vi "DigitalReadDigitalWrite.vi"() -> ()   [LabVIEW 2015]
panel:
  out "YLDRMErrorOut":errorcluster
  out "YLDRMPortOut":refnum<visa-resource-name>
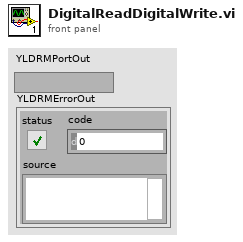
[diagram p1: front panel]
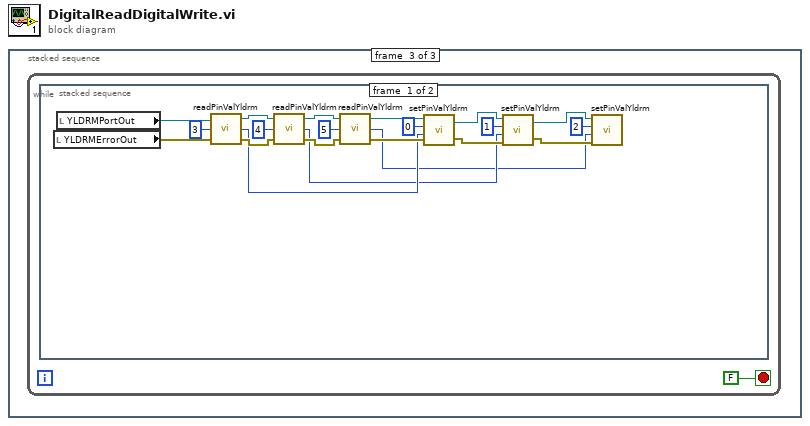
[diagram p0: block diagram]
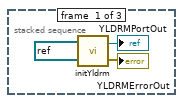
[diagram p2: hidden frame]
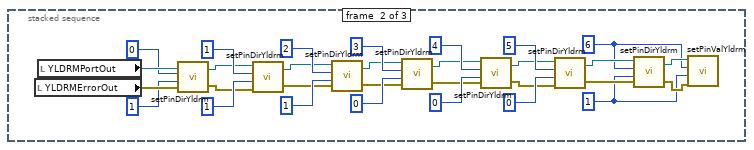
[diagram p3: hidden frame]
diagram:
  n1 = stacked-sequence {
    frame #0 {
      n2 = call "initYldrm.vi"("YLDRMPortInp"=refnum<visa-resource-name> "COM9") -> ("YLDRMPortOut"=→"YLDRMPortOut":refnum<visa-resource-name>, "YLDRMErrorOut"=→"YLDRMErrorOut":errorcluster)
    }
    frame #1 {
      w4 = u8 1 ("dir")
      w5 = u8 6 ("pin")
      n3 = local read "YLDRMErrorOut"() -> (w32:errorcluster)
      n4 = local read "YLDRMPortOut"() -> (w33:refnum<visa-resource-name>)
      n5 = call "setPinDirYldrm.vi"("YLDRMErrorInp"=w32, "dir"=u8 1, "pin"=u8 0, "YLDRMPortInp"=w33) -> ("YLDRMErrorOut"=w13:errorcluster, "YLDRMPortOut"=w19:refnum<visa-resource-name>)
      n6 = call "setPinDirYldrm.vi"("YLDRMErrorInp"=w13, "dir"=u8 1, "pin"=u8 1, "YLDRMPortInp"=w19) -> ("YLDRMErrorOut"=w12:errorcluster, "YLDRMPortOut"=w18:refnum<visa-resource-name>)
      n7 = call "setPinDirYldrm.vi"("YLDRMErrorInp"=w12, "dir"=u8 1, "pin"=u8 2, "YLDRMPortInp"=w18) -> ("YLDRMErrorOut"=w11:errorcluster, "YLDRMPortOut"=w17:refnum<visa-resource-name>)
      n8 = call "setPinDirYldrm.vi"("YLDRMErrorInp"=w11, "dir"=u8 0, "pin"=u8 3, "YLDRMPortInp"=w17) -> ("YLDRMErrorOut"=w10:errorcluster, "YLDRMPortOut"=w16:refnum<visa-resource-name>)
      n9 = call "setPinDirYldrm.vi"("YLDRMErrorInp"=w10, "dir"=u8 0, "pin"=u8 4, "YLDRMPortInp"=w16) -> ("YLDRMErrorOut"=w9:errorcluster, "YLDRMPortOut"=w15:refnum<visa-resource-name>)
      n10 = call "setPinDirYldrm.vi"("YLDRMErrorInp"=w9, "dir"=u8 0, "pin"=u8 5, "YLDRMPortInp"=w15) -> ("YLDRMErrorOut"=w8:errorcluster, "YLDRMPortOut"=w14:refnum<visa-resource-name>)
      n11 = call "setPinDirYldrm.vi"("YLDRMErrorInp"=w8, "dir"=w4, "pin"=w5, "YLDRMPortInp"=w14) -> ("YLDRMErrorOut"=w6:errorcluster, "YLDRMPortOut"=w7:refnum<visa-resource-name>)
      n12 = call "setPinValYldrm.vi"("YLDRMErrorInp"=w6, "val"=w4, "pin"=w5, "YLDRMPortInp"=w7) -> ()  [unwired: 2 out]
    }
    frame #2 {
      n13 = while {
        stop <- FALSE stop-if-true
        n14 = stacked-sequence {
          frame #0 {
            n15 = local read "YLDRMErrorOut"() -> (w54:errorcluster)
            n16 = local read "YLDRMPortOut"() -> (w55:refnum<visa-resource-name>)
            n17 = call "readPinValYldrm.vi"("YLDRMErrorInp"=w54, "pin"=u8 3, "YLDRMPortInp"=w55) -> ("YLDRMErrorOut"=w48:errorcluster, "out"=w37:u8, "YLDRMPortOut"=w50:refnum<visa-resource-name>)
            n18 = call "readPinValYldrm.vi"("YLDRMErrorInp"=w48, "pin"=u8 4, "YLDRMPortInp"=w50) -> ("YLDRMErrorOut"=w47:errorcluster, "out"=w36:u8, "YLDRMPortOut"=w49:refnum<visa-resource-name>)
            n19 = call "readPinValYldrm.vi"("YLDRMErrorInp"=w47, "pin"=u8 5, "YLDRMPortInp"=w49) -> ("YLDRMErrorOut"=w45:errorcluster, "out"=w35:u8, "YLDRMPortOut"=w46:refnum<visa-resource-name>)
            n20 = call "setPinValYldrm.vi"("YLDRMErrorInp"=w45, "val"=w37, "pin"=u8 0, "YLDRMPortInp"=w46) -> ("YLDRMErrorOut"=w40:errorcluster, "YLDRMPortOut"=w41:refnum<visa-resource-name>)
            n21 = call "setPinValYldrm.vi"("YLDRMErrorInp"=w40, "val"=w36, "pin"=u8 1, "YLDRMPortInp"=w41) -> ("YLDRMErrorOut"=w38:errorcluster, "YLDRMPortOut"=w39:refnum<visa-resource-name>)
            n22 = call "setPinValYldrm.vi"("YLDRMErrorInp"=w38, "val"=w35, "pin"=u8 2, "YLDRMPortInp"=w39) -> ()  [unwired: 2 out]
          }
          frame #1 {
          }
        }
      }
    }
  }
